vi "Create 1D Indicator Matrix.vi"(10 "Numeric Value":u8, 11 "Color":u32(colorbox)) -> (3 "Matrix":T1)   [LabVIEW 2019, in "LED Matrix Host.lvlib"]
uses:
  LED Matrix Host.lvlib
  Public/Controls/Frame.ctl
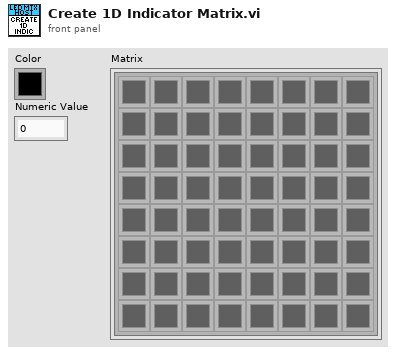
[diagram p1: front panel]
types:
  T1 = typedef "LED Matrix Host.lvlib/Frame.ctl" = cluster{"Matrix":u32[][]}
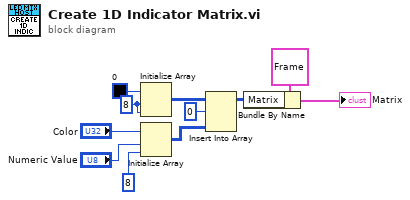
[diagram p0: block diagram]
diagram:
  w7 = 8 ("dimension size")
  n1 = Initialize Array(u32 0 ("Color Box"), w7, w7) -> (w9:u32[][])
  n2 = Initialize Array("Color", "Numeric Value", 8 ("dimension size")) -> (w4:u32[][])
  n3 = Insert Into Array(array=w9, index (row)=0, new element=w4) -> (w10:u32[][])  [unwired: 1 in]
  n4 = Bundle By Name(cluster=T1 {"Matrix"=[[0, 0, 0, 0, 0, 0, 0, 0], [16777222, 16777222, 0, 0, 0, 0, 0, 0], [0, 0, 0, 0, 0, 0, 0, 0], [0, 0, 0, 0, 0, 0, 0, 0], [0, 0, 0, 0, 0, 0, 0, 0], [0, 0, 0, 0, 0, 0, 0, 0], [0, 0, 0, 0, 0, 0, 0, 0], [16777222, 0, 0, 0, 0, 0, 0, 16777222]]} ("Matrix"), "Matrix"=w10) -> (→"Matrix":T1)
